vi "Game Info Global Variable.vi"() -> ()   [LabVIEW 2016]
panel:
  in  "P2 King Text Blue Color":i32
  in  "P2 King Text Green Color":i32
  in  "P2 King Text Red Color":i32
  in  "P1 King Text Blue Color":i32
  in  "P1 King Text Green Color":i32
  in  "P1 King Text Red Color":i32
  in  "P2 Blue Color":i32=255
  in  "P2 Green Color":i32=191
  in  "P2 Red Color":i32
  in  "P1 Blue Color":i32
  in  "P1 Green Color":i32
  in  "P1 Red Color":i32=254
  in  "Player 2 Name":string="Player 2"
  in  "Player 1 Name":string="Player 1"
  # "Player 1 Team Color:"
  # "Player 2 Team Color:"
  # "Player 1 King Text Color:"
  # "Player 2 King Text Color:"
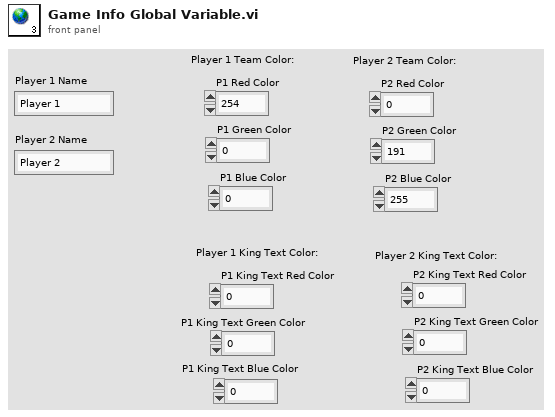
[diagram p1: front panel]
diagram:
